vi "read single temp.vi"(8 "error in (no error)":errorcluster, 11 "Thermocouples in":refnum<class "Thermocouples.lvclass">) -> (0 "error out":errorcluster, 2 "Temperature":dbl format="%0.2f", 3 "Thermocouples out":refnum<class "Thermocouples.lvclass">)   [LabVIEW 2025, in "Thermocouples.lvclass"]
uses:
  Thermocouples.lvclass
  Thermocouples.lvclass/Thermocouples.ctl
  <vilib>/DAQmx/read.llb/DAQmx Read (Analog DBL 1Chan 1Samp).vi
  <vilib>/DAQmx/miscellaneous.llb/DAQmx Fill In Error Info.vi
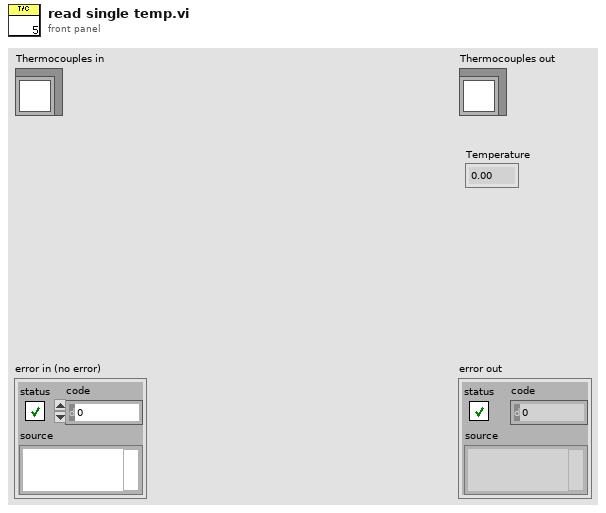
[diagram p1: front panel]
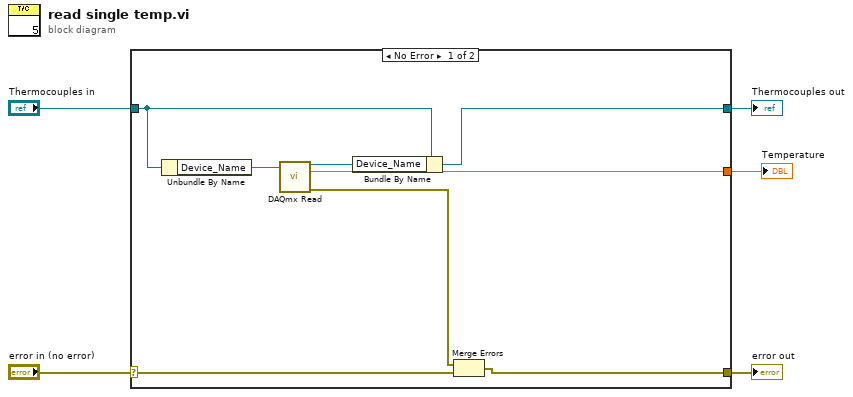
[diagram p0: block diagram]
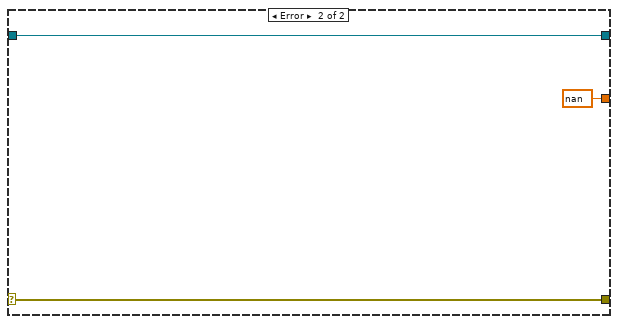
[diagram p2: hidden frame]
diagram:
  n1 = case shown="No Error" "error in (no error)" {
    selector: "error in (no error)" -> [w11 w16]
    tunnel: [w10 w16] -> w4
    tunnel: [w6 w15] -> w2
    tunnel: "Thermocouples in" -> [w8 w15]
    tunnel: [w12 nan ("data")] -> w1
    frame No Error {
      n2 = Unbundle By Name(w8) -> ("Device_Name"=w13:string)
      n3 = call-poly <vilib>:"DAQmx Read.vi"("task/channels in"=w13) -> ("task out"=w7:refnum<k21>, "data"=w12:dbl, "error out"=w9:errorcluster)  [unwired: 12 in]
      n4 = Bundle By Name(cluster=w8, "Device_Name"=w7) -> (w6:refnum<class "Thermocouples.lvclass">)
      n5 = Merge Errors(w9, w11) -> (w10:errorcluster)
    }
    frame Error {
    }
  }
  "error out" <- w4
  "Thermocouples out" <- w2
  "Temperature" <- w1
